vi "Read QoS.vi"(8 "error in (no error)":errorcluster, 11 "Subscription in":refnum<class "_Subscription.lvclass">) -> (0 "error out":errorcluster, 2 "QoS":T1, 3 "Subscription out":refnum<class "_Subscription.lvclass">)   [LabVIEW 2013, in "MQTT Server.lvlib" / "_Subscription.lvclass"]
uses:
  _Subscription.lvclass
  <vilib>/LabVIEW Open Source Project/MQTT Control Packets/Control Packets/ControlPacket/QualityOfService -- enum.ctl
  _Subscription.lvclass/_Subscription.ctl
  <vilib>/LabVIEW Open Source Project/MQTT Control Packets/Control Packets/ControlPacket/ControlPacket.lvclass
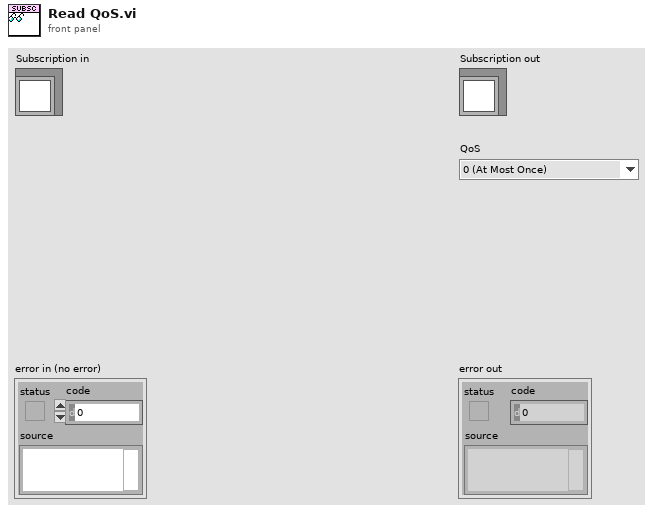
[diagram p1: front panel]
types:
  T1 = typedef "MQTT_Control_Packets.lvlib/ControlPacket.lvclass/QualityOfService -- enum.ctl" = enum16{"0 (At Most Once)", "1 (At Least Once)", "2 (Exactly Once)"}
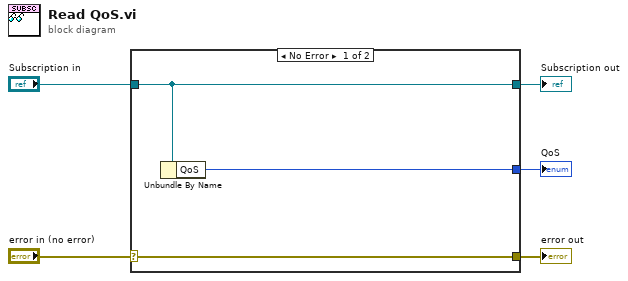
[diagram p0: block diagram]
diagram:
  n1 = case shown="No Error" "error in (no error)" {
    selector: "error in (no error)" -> [w8 w9]
    tunnel: [w8 w9] -> w4
    tunnel: [w7 w10] -> w2
    tunnel: "Subscription in" -> [w7 w10]
    tunnel: [w6 _] -> w1
    frame No Error {
      n2 = Unbundle By Name(w7) -> ("QoS"=w6:T1)
    }
    frame Error {
    }
  }
  "error out" <- w4
  "Subscription out" <- w2
  "QoS" <- w1
